vi "Init Panels.vi"(8 "error in (no error)":errorcluster, 11 "LV-Term App in":refnum<class "LV-Term App.lvclass">) -> (0 "error out":errorcluster, 3 "LV-Term App out":refnum<class "LV-Term App.lvclass">)   [LabVIEW 2020, in "LV-Term App.lvclass"]
uses:
  LV-Term App.lvclass
  LV-Term App.lvclass/LV-Term App.ctl
  <vilib>/IlluminatedG/IG OOPanel/OOPanel/Manager/Manager.lvclass
  Terminal/Terminal/Terminal.lvclass
  C:/Program Files (x86)/National Instruments/LabVIEW 2020/vi.lib/IlluminatedG/IG OOPanel/OOPanel/Panel/Panel.lvclass
  C:/dev/IlluminatedG/lv-stream-terminal/Terminal/Terminal/Terminal.lvclass
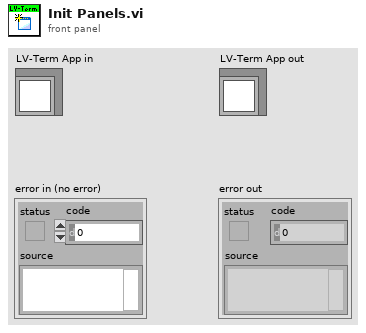
[diagram p1: front panel]
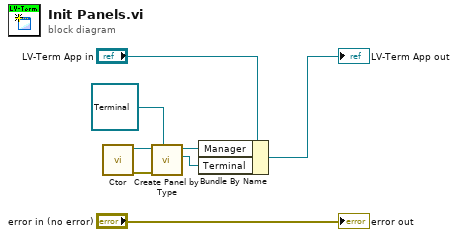
[diagram p0: block diagram]
diagram:
  n1 = call <vilib>:"Ctor.vi"() -> ("error out"=w5:errorcluster, "Manager out"=w7:refnum<class "Manager.lvclass">)  [unwired: 10 in]
  n2 = call <vilib>:"Create Panel by Type.vi"("Panel Type"=refnum<class "Terminal.lvclass"> refnum ("Terminal.lvlib:Terminal.lvclass"), "error in (no error)"=w5, "Manager in"=w7) -> ("Panel"=w3:refnum<class "Terminal.lvclass">, "Manager out"=w4:refnum<class "Manager.lvclass">)  [unwired: 6 in, 1 out]
  n3 = Bundle By Name(cluster="LV-Term App in", "Manager"=w4, "Terminal"=w3) -> (→"LV-Term App out":refnum<class "LV-Term App.lvclass">)
  "error out" <- "error in (no error)"
